vi "HRM-AQN-Set_waveform_size.vi"(9 "samples [s]":i32, 10 "Raw collected data":waveform(dbl), 11 "Raw data in":waveform(dbl)) -> (2 "Raw collected data out":waveform(dbl))   [LabVIEW 2020]
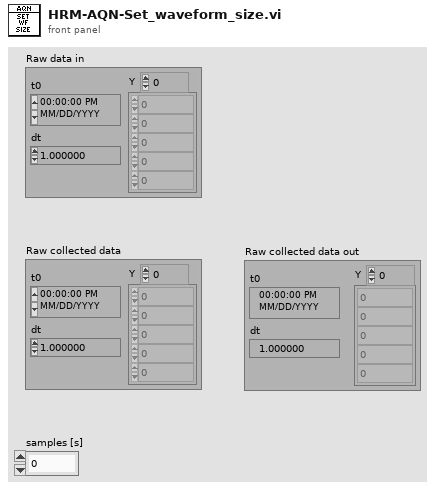
[diagram p1: front panel]
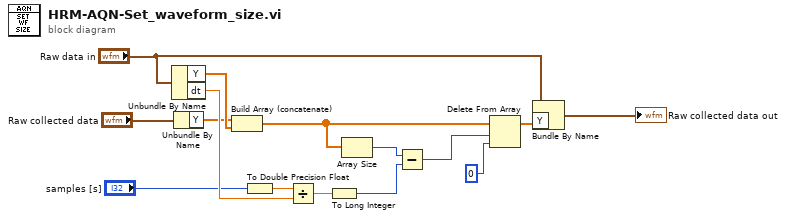
[diagram p0: block diagram]
diagram:
  n1 = Unbundle By Name("Raw data in") -> ("Y"=w3:dbl[], "dt"=w10:dbl)
  n2 = Unbundle By Name("Raw collected data") -> ("Y"=w2:dbl[])
  n3 = Build Array (concatenate)(w2, w3) -> (w12:dbl[])
  n4 = To Double Precision Float(number="samples [s]") -> (double precision float=w9:dbl)
  n5 = Divide(x=w9, y=w10) -> (x/y=w11:dbl)
  n6 = To Long Integer(number=w11) -> (32bit integer=w14:i32)
  n7 = Array Size(array=w12) -> (size(s)=w13:i32)
  n8 = Subtract(x=w13, y=w14) -> (x-y=w15:i32)
  n9 = Delete From Array(array=w12, length=w15, index=0) -> (array with subset deleted=w6:dbl[])  [unwired: 1 out]
  n10 = Bundle By Name(cluster="Raw data in", "Y"=w6) -> (→"Raw collected data out":waveform(dbl))
